vi "max and min values.vi"() -> ()   [LabVIEW 2025]
panel:
  out "min number":dbl
  out "max number":dbl
  in  "Array":dbl[](array[numeric])
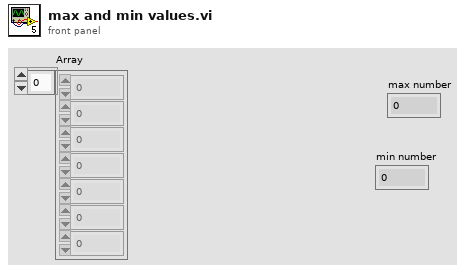
[diagram p1: front panel]
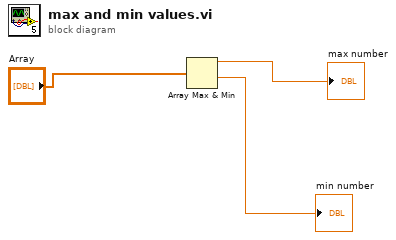
[diagram p0: block diagram]
diagram:
  n1 = Array Max & Min(array="Array") -> (max value=→"max number":dbl, min value=→"min number":dbl)  [unwired: 2 out]
